vi "SNED_FLOAT_T_CHANNEL_V_S_BEIFEN.vi"(1 "数据":dbl, 2 "字符":string, 3 "通道":string, 4 "T":string) -> (0 "处理之后的数据":string)   [LabVIEW 2014]
panel:
  out "Numeric":u8
  out "第一个校验数据":u8
  out "String 2":string
  out "4":u8
  out "3":u8
  out "2":u8
  out "1":u8
  out "String":string
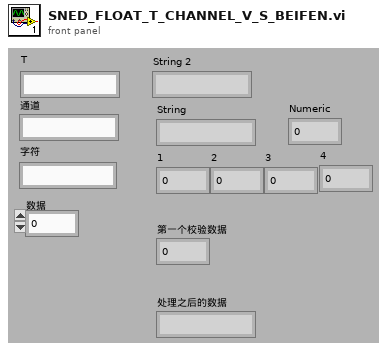
[diagram p1: front panel]
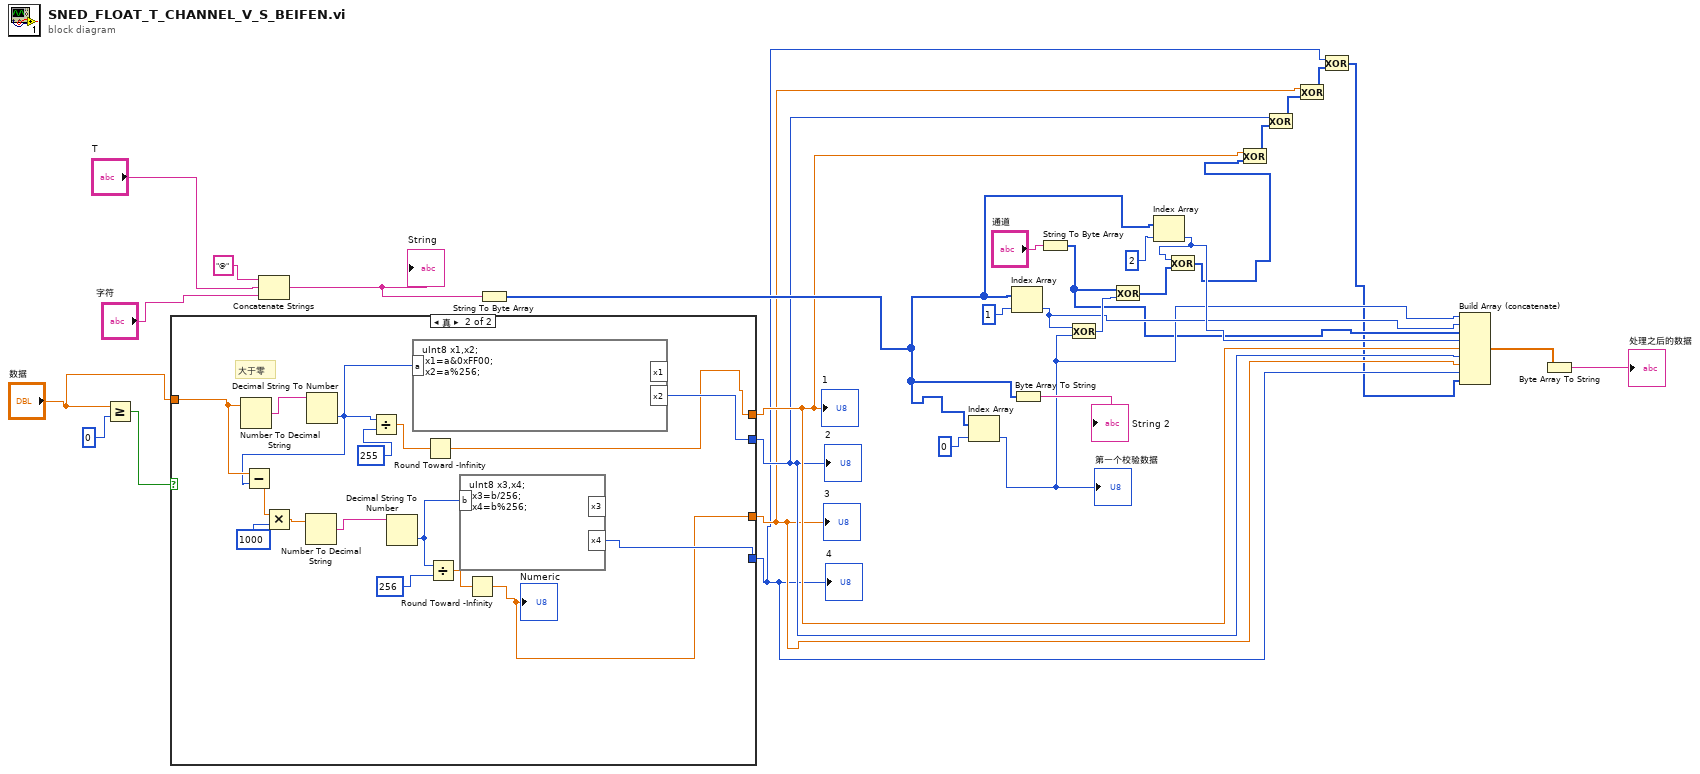
[diagram p0: block diagram]
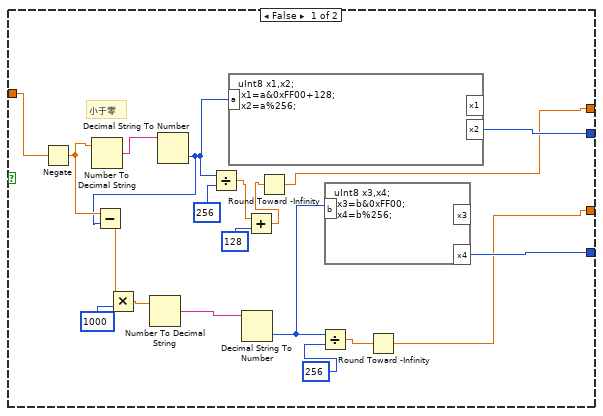
[diagram p2: hidden frame]
diagram:
  n1 = Greater Or Equal?(x="数据", y=0) -> (x >= y?=w5:bool)
  n2 = case shown="真" w5 {
    tunnel: "数据" -> [w41 w61]
    tunnel: [w39 w50] -> w10
    tunnel: [w43 w60] -> w9
    tunnel: [w35 w54] -> w8
    tunnel: [w42 w59] -> w7
    frame False {
      # "小于零"
      n3 = Negate(x=w41) -> (-x=w44:dbl)
      n4 = Number To Decimal String(number=w44) -> (decimal integer string=w45:string)  [unwired: 1 in]
      n5 = Decimal String To Number(string=w45) -> (number=w40:i32)  [unwired: 2 in, 1 out]
      n6 = Subtract(x=w44, y=w40) -> (x-y=w48:dbl)
      n7 = Multiply(x=w48, y=1000) -> (x*y=w46:dbl)
      n8 = Number To Decimal String(number=w46) -> (decimal integer string=w49:string)  [unwired: 1 in]
      n9 = Divide(x=w40, y=256) -> (x/y=w33:dbl)
      n10 = formula code="uInt8 x1,x2;\n x1=a&0xFF00+128;\n x2=a%256;"("a"=w40) -> ("x2"=w43:u8)  [unwired: 1 out]
      n11 = Decimal String To Number(string=w49) -> (number=w37:i32)  [unwired: 2 in, 1 out]
      n12 = Add(x=w33, y=128) -> (x+y=w31:dbl)
      n13 = Round Toward -Infinity(1:w31) -> (0:w39:dbl)
      n14 = Divide(x=w37, y=256) -> (x/y=w38:dbl)
      n15 = formula code="uInt8 x3,x4;\n x3=b&0xFF00;\n x4=b%256;"("b"=w37) -> ("x4"=w42:u8)  [unwired: 1 out]
      n16 = Round Toward -Infinity(1:w38) -> (0:w35:dbl)
    }
    frame True {
      # "大于零"
      n17 = Number To Decimal String(number=w61) -> (decimal integer string=w62:string)  [unwired: 1 in]
      n18 = Decimal String To Number(string=w62) -> (number=w53:i32)  [unwired: 2 in, 1 out]
      n19 = Subtract(x=w61, y=w53) -> (x-y=w65:dbl)
      n20 = Multiply(x=w65, y=1000) -> (x*y=w63:dbl)
      n21 = Number To Decimal String(number=w63) -> (decimal integer string=w55:string)  [unwired: 1 in]
      n22 = Divide(x=w53, y=255) -> (x/y=w51:dbl)
      n23 = Decimal String To Number(string=w55) -> (number=w58:i32)  [unwired: 2 in, 1 out]
      n24 = formula code="uInt8 x1,x2;\n x1=a&0xFF00;\n x2=a%256;"("a"=w53) -> ("x2"=w60:u8)  [unwired: 1 out]
      n25 = Round Toward -Infinity(1:w51) -> (0:w50:dbl)
      n26 = Divide(x=w58, y=256) -> (x/y=w56:dbl)
      n27 = formula code="uInt8 x3,x4;\n x3=b/256;\n x4=b%256;"("b"=w58) -> ("x4"=w59:u8)  [unwired: 1 out]
      n28 = Round Toward -Infinity(1:w56) -> (0:w54:dbl)
      "Numeric" <- w54
    }
  }
  "1" <- w10
  "2" <- w9
  "3" <- w8
  "4" <- w7
  n29 = Concatenate Strings("@", "T", "字符") -> (w29:string)
  "String" <- w29
  n30 = String To Byte Array(string=w29) -> (unsigned byte array=w16:u8[])
  n31 = Index Array(array=w16, index=0) -> (element=w12:u8)
  "第一个校验数据" <- w12
  n32 = Index Array(array=w16, index=1) -> (element=w13:u8)
  n33 = Byte Array To String(unsigned byte array=w16) -> (string=→"String 2":string)
  n34 = String To Byte Array(string="通道") -> (unsigned byte array=w3:u8[])
  n35 = Exclusive Or(1:w12, 2:w13) -> (0:w18:u8)
  n36 = Exclusive Or(1:w18, 2:w3) -> (0:w15:u8[])
  n37 = Index Array(array=w16, index=2) -> (element=w14:u8)
  n38 = Exclusive Or(1:w15, 2:w14) -> (0:w11:u8[])
  n39 = Exclusive Or(1:w11, 2:w10) -> (0:w25:i32[])
  n40 = Exclusive Or(1:w25, 2:w9) -> (0:w24:i32[])
  n41 = Exclusive Or(1:w24, 2:w8) -> (0:w23:i32[])
  n42 = Exclusive Or(1:w23, 2:w7) -> (0:w2:i32[])
  n43 = Build Array (concatenate)(w12, w13, w3, w14, w10, w9, w8, w7, w2) -> (w22:dbl[])
  n44 = Byte Array To String(unsigned byte array=w22) -> (string=→"处理之后的数据":string)
